vi "WatchDogSam.vi"(11 "watchdogID":u64) -> ()   [LabVIEW 2014]
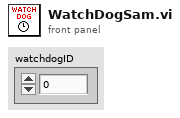
[diagram p1: front panel]
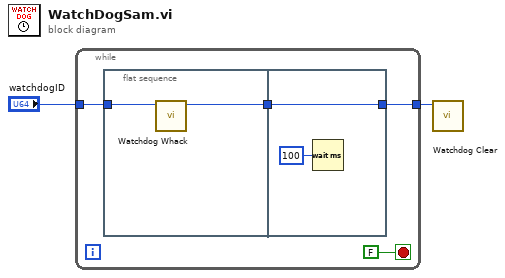
[diagram p0: block diagram]
diagram:
  n1 = while {
    tunnel: "watchdogID" -> [w6]
    tunnel: [w5] -> w2
    stop <- FALSE stop-if-true
    n2 = flat-sequence {
      tunnel: w6 -> [w8]
      tunnel: [w7] -> w4
      tunnel: [w9] -> w5
      tunnel: w4 -> [w9]
      frame #0 {
        n3 = call <vilib>:"Watchdog Whack.vi"("watchdogID in"=w8) -> ("watchdogID out"=w7:u64)  [unwired: 4 in, 2 out]
      }
      frame #1 {
        n4 = Wait (ms)(milliseconds to wait=u32 100) -> ()  [unwired: 1 out]
      }
    }
  }
  n5 = call <vilib>:"Watchdog Clear.vi"("watchdogID in"=w2) -> ()  [unwired: 6 in, 1 out]
